vi "hidSPD Setup Signal Board.vi"(8 "error in (no error)":errorcluster, 10 "hidSPD Signal Setup Report":T1={"strob_gain"=-1, "receive_gain"=-1, "positive_bias"=-1, "negative_bias"=-1, "deadtime"=-1, "insensitivity"=-1, "deadtime_strobe"=-1, "dt_on"=-1, "frequency"=-1, "pllpwr"=-1, "rvset"=-1, "dvset"=-1}, 11 "spdDevSession in":T2={"spdRef"=0, "connected"=FALSE, "spdName"="", "specification"={"diod case"=enum."default", "type"=enum."Unknown", "frequency"=enum."Unknown"}, "hidSPD.Controller"={"TSet"=0.0, "HV_bias"=0.0, "DDS_stb_code"=0}, "hidSPD.Sturtup Values"={"TSet"=0.0, "HV_bias"=0.0, "DDS_stb_code"=0}} {"hidSPD.Sturtup Values"."HV_bias" format="%#_6p, V"; "hidSPD.Sturtup Values"."TSet" format="%#_6p, DegC"; "hidSPD.Controller"."HV_bias" format="%#_6p, V"; "hidSPD.Controller"."TSet" format="%#_6p, DegC"}) -> (0 "error out":errorcluster, 3 "spdDevSession out":T2={"spdRef"=0, "connected"=FALSE, "spdName"="", "specification"={"diod case"=enum."default", "type"=enum."Unknown", "frequency"=enum."Unknown"}, "hidSPD.Controller"={"TSet"=0.0, "HV_bias"=0.0, "DDS_stb_code"=0}, "hidSPD.Sturtup Values"={"TSet"=0.0, "HV_bias"=0.0, "DDS_stb_code"=0}} {"hidSPD.Sturtup Values"."HV_bias" format="%#_6p, V"; "hidSPD.Sturtup Values"."TSet" format="%#_6p, DegC"; "hidSPD.Controller"."HV_bias" format="%#_6p, V"; "hidSPD.Controller"."TSet" format="%#_6p, DegC"})   [LabVIEW 2018, in "hidSPDLibForLabView.lvlib"]
uses:
  hidSPDLibForLabView.lvlib
  hidSPD Controls/hidSPD Device Session.ctl
  hidSPD Controls/hidSPD.SPD specification.ctl
  hidSPD Controls/hidSPD SPD Diod Case.ctl
  hidSPD Controls/hidSPD SPD Type.ctl
  hidSPD Controls/hidSPD.STB Frequency.ctl
  hidSPD Controls/hidSPD Controller.ctl
  hidSPD Controls/hidSPD Controller Signal Report.ctl
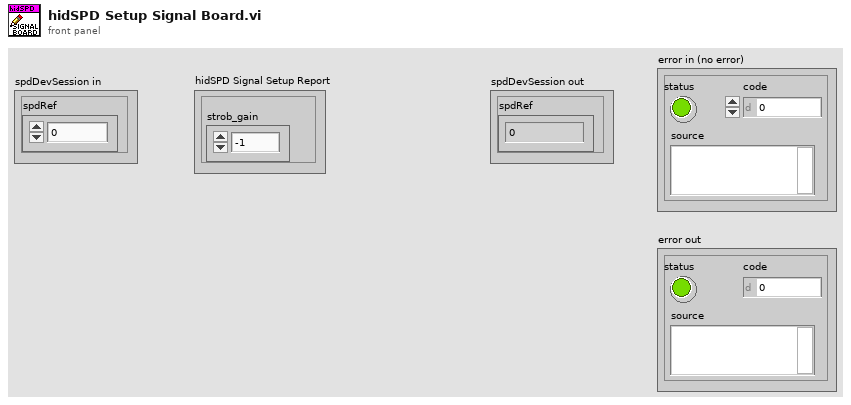
[diagram p1: front panel]
types:
  T1 = typedef "hidSPDLibForLabView.lvlib/hidSPD Controller Signal Report.ctl" = cluster{"strob_gain":i8, "receive_gain":i8, "positive_bias":i32, "negative_bias":i32, "deadtime":i16, "insensitivity":i16, "deadtime_strobe":i8, "dt_on":i8, "frequency":i16, "pllpwr":i8, "rvset":i16, "dvset":i16}
  T2 = typedef "hidSPDLibForLabView.lvlib/hidSPD Device Session.ctl" = cluster{"spdRef":u64, "connected":bool, "spdName":string, "specification":T3, "hidSPD.Controller":T7, "hidSPD.Sturtup Values":T7}
  T3 = typedef "hidSPDLibForLabView.lvlib/hidSPD.SPD specification.ctl" = cluster{"diod case":T4, "type":T5, "frequency":T6}
  T4 = typedef "hidSPDLibForLabView.lvlib/hidSPD SPD Diod Case.ctl" = enum16{"Unknown", "default", "butterfly"}
  T5 = typedef "hidSPDLibForLabView.lvlib/hidSPD SPD Type.ctl" = enum16{"Unknown", "Free Run", "Gate"}
  T6 = typedef "hidSPDLibForLabView.lvlib/hidSPD.STB Frequency.ctl" = enum16{"Unknown", "312", "1250"}
  T7 = typedef "hidSPDLibForLabView.lvlib/hidSPD Controller.ctl" = cluster{"TSet":sgl, "HV_bias":sgl, "DDS_stb_code":u16}
  T8 = enum16{"big-endian, network order", "native, host order", "little-endian"}
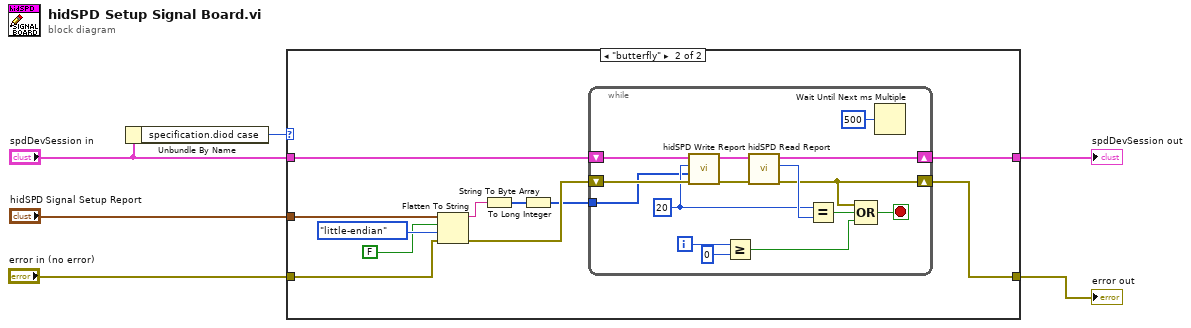
[diagram p0: block diagram]
diagram:
  n1 = Unbundle By Name("spdDevSession in") -> ("specification.diod case"=w4:T4)
  n2 = case shown="\"butterfly\"" w4 {
    tunnel: "spdDevSession in" -> [w8 w19]
    tunnel: [w8 w18] -> w6
    tunnel: "error in (no error)" -> [w7 w15]
    tunnel: "hidSPD Signal Setup Report" -> [_ w12]
    tunnel: [w7 w9] -> w1
    frame "Unknown", Default {
    }
    frame "butterfly" {
      n3 = Flatten To String(anything=w12, prepend array or string size? (T)=FALSE, byte order (0:big-endian, network order)=T8."little-endian", error in (no error)=w15) -> (data string=w17:string, error out=w11:errorcluster)  [unwired: 1 out]
      n4 = String To Byte Array(string=w17) -> (unsigned byte array=w16:u8[])
      n5 = To Long Integer(number=w16) -> (32bit integer=w10:i32[])
      n6 = while {
        shift-right: [w34] -> w18
        shift-left: w19 -> [w28]
        shift-right: [w30] -> w9
        shift-left: w11 -> [w27]
        tunnel: w10 -> [w20]
        i -> [w23]
        stop <- w29 stop-if-true
        w26 = 20 ("cmd")
        n7 = call "hidSPD Write Report.vi"("error in (no error)"=w27, "data"=w20, "cmd"=w26, "spdDevSession in"=w28) -> ("error out"=w25:errorcluster, "spdDevSession out"=w24:T2)  [unwired: 6 in]
        n8 = Greater Or Equal?(x=w23, y=0) -> (x >= y?=w21:bool)
        n9 = call "hidSPD Read Report.vi"("error in (no error)"=w25, "spdDevSession in"=w24) -> ("error out"=w30:errorcluster, "cmd"=w32:i32, "spdDevSession out"=w34:T2)  [unwired: 6 in, 1 out]
        n10 = Equal?(x=w26, y=w32) -> (x = y?=w31:bool)
        n11 = Compound Arithmetic op=OR(w30, w31, w21) -> (w29:bool)
        n12 = Wait Until Next ms Multiple(millisecond multiple=u32 500) -> ()  [unwired: 1 out]
      }
    }
  }
  "error out" <- w1
  "spdDevSession out" <- w6
